vi "Init Scope.vi"(1 "Timeout (ms)":u32=2000, 4 "Scope Control References":T2, 5 "Repetitive Signal":bool, 6 "Reset Settings":bool, 7 "error in (no error)":errorcluster, 8 "Scope Config on Startup":enum16{"PC->Scope", "Scope->PC"}(ring)=enum."Scope->PC", 9 "Scope Model":T1=enum."Tek TDS 694C", 10 "Scope Address":refnum<visa-resource-name>) -> (0 "error out":errorcluster, 2 "Instrument ID":string, 3 "reference out":refnum<visa-resource-name>)   [LabVIEW 2020]
uses:
  Typedefs/Scope Control References Control.ctl
  Typedefs/Scope Models.ctl
  730dcbdf-4df6-4714-a0fe-e75e7198162a.vi
  7d0b5108-51c8-4697-949d-e607a969f50b.vi
  <instrlib>/tktds7xx/tktds7xx.llb/TKTDS 7XX Trigger Mode/Holdoff.vi
  <vilib>/Comparison/Equal/Equal Functor/Equal Functor.lvclass
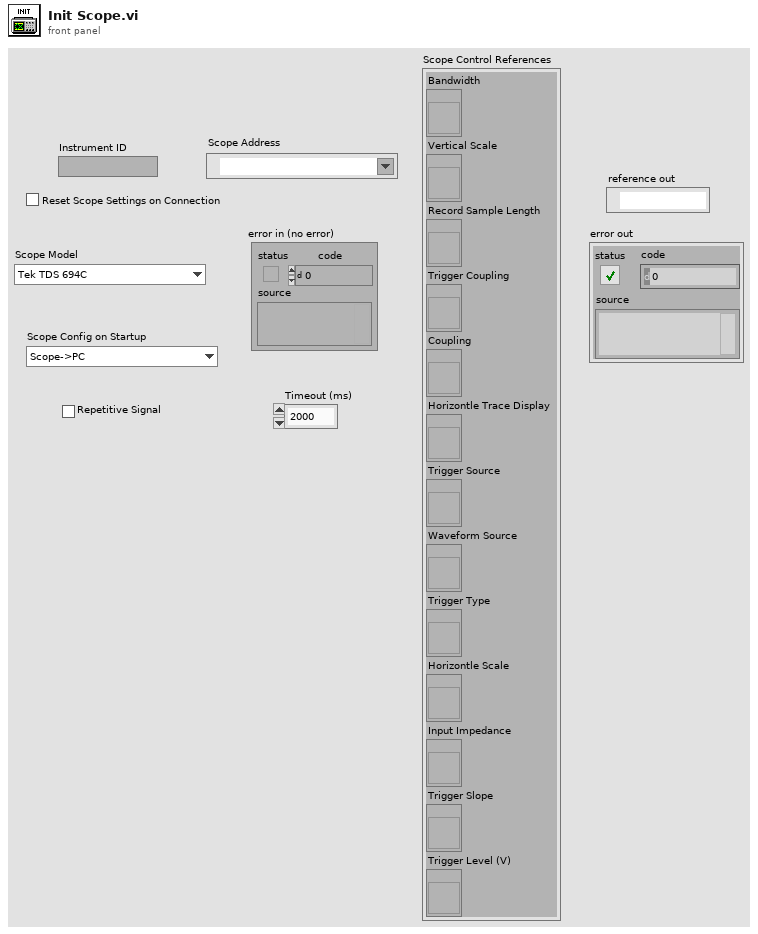
[diagram p1: front panel]
types:
  T1 = typedef "Scope Models.ctl" = enum16{"Tek TDS 684A/B/C", "Tek TDS 694C", "Tek TDS 744/A", "Tek TDS 754A/C/D", "Tek TDS 784A/C/D"}
  T2 = typedef "Scope Control References Control.ctl" = cluster{"Bandwidth":refnum<vi>, "Vertical Scale":refnum<vi>, "Record Sample Length":refnum<vi>, "Trigger Coupling":refnum<vi>, "Coupling":refnum<vi>, "Horizontle Trace Display":refnum<vi>, "Trigger Source":refnum<vi>, "Waveform Source":refnum<vi>, "Trigger Type":refnum<vi>, "Horizontle Scale":refnum<vi>, "Input Impedance":refnum<vi>, "Trigger Slope":refnum<vi>, "Trigger Level (V)":refnum<vi>}
  T3 = cluster{"delay mode (runs after:0)":i32, "delay scaling (50micros/div:16)":i32, "delay events (2)":ext, "delay by (time:0)":i32, "delay time (16.0E-9)":ext}
  T4 = cluster{"Attenuation (Multiplier)":dbl, "Scale (V/Div)":dbl, "Position (V)":dbl, "Offset (V)":dbl, "Coupling":u16, "Impedance":i32, "Bandwidth":i32, "Deskew (s)":dbl}
  T5 = cluster{"Horizontal Mode\n(main only:0)":i32, "Record Length":i32, "Main Scaling (s/Div)":dbl, "Delay Scaling (s/Div)":dbl, "Delay Time (s)":dbl, "Horizontal Position (%)":dbl, "Trigger Position (%)":dbl}
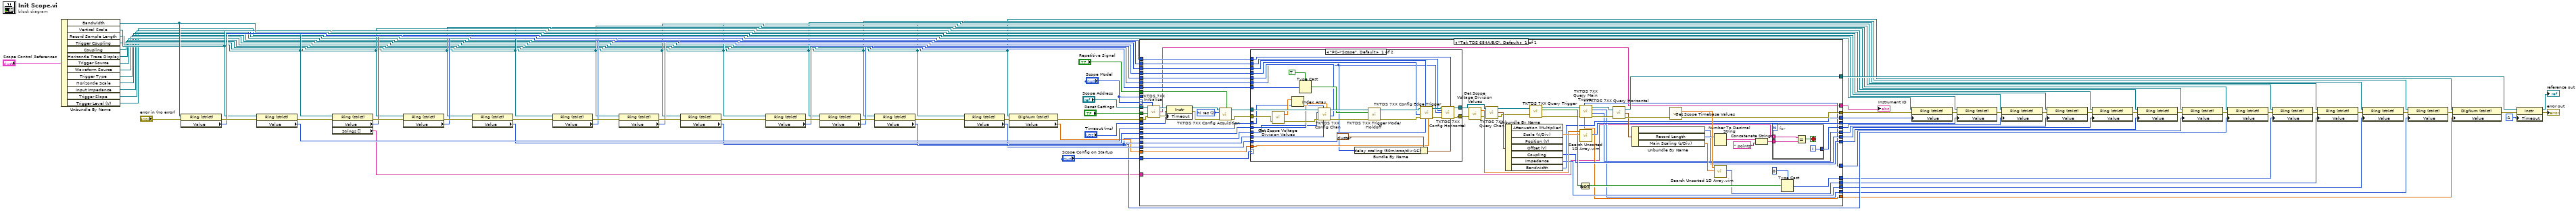
[diagram p0: block diagram]
diagram:
  n1 = Unbundle By Name("Scope Control References") -> ("Bandwidth"=w32:refnum<vi>, "Vertical Scale"=w31:refnum<vi>, "Record Sample Length"=w30:refnum<vi>, "Trigger Coupling"=w29:refnum<vi>, "Coupling"=w28:refnum<vi>, "Horizontle Trace Display"=w27:refnum<vi>, "Trigger Source"=w26:refnum<vi>, "Waveform Source"=w25:refnum<vi>, "Trigger Type"=w24:refnum<vi>, "Horizontle Scale"=w23:refnum<vi>, "Input Impedance"=w22:refnum<vi>, "Trigger Slope"=w21:refnum<vi>, "Trigger Level (V)"=w20:refnum<vi>)
  n2 = property on="Property Node" class="Ring (strict)"(reference=w32, error in="error in (no error)") -> (error out=w75:errorcluster, "Value"=w62:u16)  [unwired: 1 out]
  n3 = property on="Property Node" class="Ring (strict)"(reference=w31, error in=w75) -> (error out=w74:errorcluster, "Value"=w63:u16)  [unwired: 1 out]
  n4 = property on="Property Node" class="Ring (strict)"(reference=w30, error in=w74) -> (error out=w73:errorcluster, "Value"=w54:i32, "Strings []"=w6:string[])  [unwired: 1 out]
  n5 = property on="Property Node" class="Ring (strict)"(reference=w29, error in=w73) -> (error out=w72:errorcluster, "Value"=w56:i32)  [unwired: 1 out]
  n6 = property on="Property Node" class="Ring (strict)"(reference=w28, error in=w72) -> (error out=w71:errorcluster, "Value"=w61:u16)  [unwired: 1 out]
  n7 = property on="Property Node" class="Ring (strict)"(reference=w27, error in=w71) -> (error out=w70:errorcluster, "Value"=w53:i32)  [unwired: 1 out]
  n8 = property on="Property Node" class="Ring (strict)"(reference=w26, error in=w70) -> (error out=w69:errorcluster, "Value"=w55:u16)  [unwired: 1 out]
  n9 = property on="Property Node" class="Ring (strict)"(reference=w25, error in=w69) -> (error out=w68:errorcluster, "Value"=w12:u16)  [unwired: 1 out]
  n10 = property on="Property Node" class="Ring (strict)"(reference=w24, error in=w68) -> (error out=w67:errorcluster, "Value"=w59:u16)  [unwired: 1 out]
  n11 = property on="Property Node" class="Ring (strict)"(reference=w23, error in=w67) -> (error out=w66:errorcluster, "Value"=w52:i32)  [unwired: 1 out]
  n12 = property on="Property Node" class="Ring (strict)"(reference=w22, error in=w66) -> (error out=w65:errorcluster, "Value"=w60:u16)  [unwired: 1 out]
  n13 = property on="Property Node" class="Ring (strict)"(reference=w21, error in=w65) -> (error out=w64:errorcluster, "Value"=w58:i32)  [unwired: 1 out]
  n14 = property on="Property Node" class="DigNum (strict)"(reference=w20, error in=w64) -> (error out=w3:errorcluster, "Value"=w57:dbl)  [unwired: 1 out]
  n15 = case shown="\"Tek TDS 684A/B/C\", Default" "Scope Model" {
    selector: "Scope Model" -> [w81]
    tunnel: "Scope Model" -> [_]
    tunnel: "Repetitive Signal" -> [w144]
    tunnel: "Scope Config on Startup" -> [w143]
    tunnel: "Scope Address" -> [w139]
    tunnel: "Reset Settings" -> [w138]
    tunnel: w63 -> [w137]
    tunnel: w62 -> [w136]
    tunnel: w61 -> [w135]
    tunnel: w60 -> [w134]
    tunnel: w59 -> [w133]
    tunnel: w58 -> [w132]
    tunnel: w57 -> [w131]
    tunnel: w56 -> [w130]
    tunnel: w55 -> [w129]
    tunnel: w54 -> [w128]
    tunnel: w53 -> [w127]
    tunnel: w52 -> [w126]
    tunnel: [w103] -> w49
    tunnel: "Timeout (ms)" -> [w102]
    tunnel: [w101] -> w35
    tunnel: [w100] -> w19
    tunnel: [w99] -> w18
    tunnel: [w98] -> w17
    tunnel: [w97] -> w16
    tunnel: [w96] -> w15
    tunnel: [w95] -> w14
    tunnel: [w94] -> w13
    tunnel: w12 -> [w93]
    tunnel: [w92] -> w11
    tunnel: [w91] -> w10
    tunnel: [w90] -> w9
    tunnel: [w89] -> w8
    tunnel: [w88] -> w7
    tunnel: w6 -> [w87]
    tunnel: w3 -> [w83]
    tunnel: [w80] -> w1
    frame "Tek TDS 684A/B/C", Default {
      w145 = 2 items=["sample", "peak detect", "hi res", "envelope", "average"] ("acqusition mode (0:sample)")
      n16 = call <instrlib>:"TKTDS 7XX Initialize.vi"("instrument descriptor (GPIB::2)"=w139, "reset"=w138, "error in (no error)"=w83, "model"=w81) -> ("VISA session"=w86:refnum<visa-resource-name>, "Instrument ID"=w80:string, "error out"=w142:errorcluster)  [unwired: 1 in]
      n17 = property class="Instr"(reference=w86, error in=w142, "Timeout"=w102) -> (reference out=w85:refnum<visa-resource-name>, error out=w141:errorcluster)
      n18 = call <instrlib>:"TKTDS 7XX Config Acquisition.vi"("error in (no error)"=w141, "acqusition mode (0:sample)"=w145, "VISA session"=w85, "repetitive signal (T:on)"=w144) -> ("error out"=w82:errorcluster, "dup VISA session"=w140:refnum<visa-resource-name>)  [unwired: 4 in]
      n19 = case shown="\"PC->Scope\", Default" w143 {
        tunnel: w82 -> [w173 w181]
        tunnel: w140 -> [w170 w180]
        tunnel: w137 -> [w165 _]
        tunnel: w136 -> [w164 _]
        tunnel: w135 -> [w163 _]
        tunnel: w93 -> [w159 _]
        tunnel: w134 -> [w162 _]
        tunnel: w133 -> [w161 _]
        tunnel: w132 -> [w158 _]
        tunnel: w131 -> [w157 _]
        tunnel: w130 -> [w156 _]
        tunnel: w129 -> [w155 _]
        tunnel: w128 -> [w154 _]
        tunnel: w127 -> [w153 _]
        tunnel: w126 -> [w152 _]
        tunnel: [w151 w181] -> w105
        tunnel: [w150 w180] -> w104
        frame "PC->Scope", Default {
          n20 = call "Get Scope Voltage Division Values.vi"("error in (no error)"=w173) -> ("error out"=w167:errorcluster, "Volts Per Division Values Array"=w166:dbl[])  [unwired: 1 in]
          n21 = Index Array(array=w166, index=w165) -> (element=w174:dbl)
          n22 = Type Cast(type=TRUE, x=w161) -> (*(type *) &x=w175:bool)
          n23 = call <instrlib>:"TKTDS 7XX Config Chan.vi"("bandwidth (20MHz:0)"=w164, "scaling (1.0)"=w174, "impedance (50ohms:0)"=w162, "coupling (DC:1)"=w163, "error in (no error)"=w167, "channel to set (ch1:0)"=w159, "VISA session"=w170) -> ("error out"=w160:errorcluster, "dup VISA session"=w177:refnum<visa-resource-name>)  [unwired: 2 in, 1 out]
          n24 = Bundle By Name(cluster=T3 {"delay mode (runs after:0)"=0, "delay scaling (50micros/div:16)"=18, "delay events (2)"=2.0, "delay by (time:0)"=0, "delay time (16.0E-9)"=1.6e-08}, "delay scaling (50micros/div:16)"=w152) -> (w178:T3)
          n25 = call "TKTDS 7XX Trigger Mode/Holdoff.vi"("error in (no error)"=w160, "trigger mode (T:auto)"=w175, "VISA session"=w177) -> ("error out"=w172:errorcluster, "dup VISA session"=w169:refnum<visa-resource-name>)  [unwired: 6 in, 1 out]
          n26 = call <instrlib>:"TKTDS 7XX Config Edge Trigger.vi"("voltage level"=w157, "trigger slope (pos:0)"=w158, "trigger coupling (DC:1)"=w156, "error in (no error)"=w172, "trigger source (ch1:0)"=w155, "VISA session"=w169) -> ("error out"=w171:errorcluster, "dup VISA session"=w168:refnum<visa-resource-name>)  [unwired: 4 in]
          n27 = call <instrlib>:"TKTDS 7XX Config Horizontal.vi"("VISA session"=w168, "record length (500:0)"=w154, "horizontal mode\n(main only:0)"=w153, "main scaling\n(500ps:1)"=w152, "error in (no error)"=w171, 14:w178) -> ("dup VISA session"=w150:refnum<visa-resource-name>, "error out"=w151:errorcluster)  [unwired: 8 in]
        }
        frame "Scope->PC" {
        }
      }
      n28 = call "Get Scope Voltage Division Values.vi"("error in (no error)"=w105) -> ("error out"=w84:errorcluster, "Volts Per Division Values Array"=w125:dbl[])  [unwired: 1 in]
      n29 = call <instrlib>:"TKTDS 7XX Query Chan.vi"("error in (no error)"=w84, "VISA session"=w104) -> ("error out"=w111:errorcluster, "Channel Settings Cluster"=w115:T4, "dup VISA session"=w108:refnum<visa-resource-name>)  [unwired: 1 in]
      n30 = Unbundle By Name(w115) -> ("Scale (V/Div)"=w118:dbl, "Coupling"=w96:u16, "Impedance"=w90:i32, "Bandwidth"=w100:i32)  [unwired: 3 out]
      n31 = call <instrlib>:"TKTDS 7XX Query Trigger.vi"("VISA session"=w108, "error in (no error)"=w111) -> ("dup VISA session"=w109:refnum<visa-resource-name>, "Auto Trigger?"=w116:bool, "error out"=w112:errorcluster)  [unwired: 1 out]
      n32 = Not(x=w116) -> (.not. x?=w117:bool)
      n33 = call <instrlib>:"TKTDS 7XX Query Main Trigger.vi"("error in (no error)"=w112, "VISA session"=w109) -> ("error out"=w113:errorcluster, "Trigger Coupling"=w97:i32, "Trigger Slope"=w89:i32, "dup VISA session"=w110:refnum<visa-resource-name>, "Trigger Level (V)"=w88:dbl, "Trigger Source"=w94:i32)  [unwired: 2 in]
      n34 = call "Search Unsorted 1D Array.vim"("element"=w118, "unsorted 1D array"=w125) -> ("index of element"=w99:i32)  [unwired: 9 in]
      n35 = call <instrlib>:"TKTDS 7XX Query Horizontal.vi"("VISA session"=w110, "error in (no error)"=w113) -> ("dup VISA session"=w103:refnum<visa-resource-name>, "Horizontal Settings"=w114:T5, "error out"=w124:errorcluster)
      n36 = Unbundle By Name(w114) -> ("Horizontal Mode\n(main only:0)"=w95:i32, "Record Length"=w120:i32, "Main Scaling (s/Div)"=w119:dbl)
      n37 = call "Get Scope Timebase Values.vi"("error in (no error)"=w124) -> ("error out"=w101:errorcluster, "Timebase Values Array"=w123:dbl[])  [unwired: 1 in]
      n38 = Number To Decimal String(number=w120) -> (decimal integer string=w121:string)  [unwired: 1 in]
      n39 = call "Search Unsorted 1D Array.vim"("element"=w119, "unsorted 1D array"=w123) -> ("index of element"=w91:i32)  [unwired: 9 in]
      n40 = Concatenate Strings(w121, " points" ("string")) -> (w122:string)
      n41 = for {
        tunnel: w87 -> [w149] mode=indexing
        tunnel: w122 -> [w148]
        tunnel: [w146] -> w98
        i -> [w146]
        stop <- w147 stop-if-true
        n42 = Equal?(x=w149, y=w148) -> (x = y?=w147:bool)
      }
      n43 = Type Cast(type=0, x=w117) -> (*(type *) &x=w92:i32)
    }
  }
  "Instrument ID" <- w1
  n44 = property on="Property Node" class="Ring (strict)"(reference=w32, error in=w35, "Value"=w19) -> (error out=w47:errorcluster)  [unwired: 1 out]
  n45 = property on="Property Node" class="Ring (strict)"(reference=w31, error in=w47, "Value"=w18) -> (error out=w46:errorcluster)  [unwired: 1 out]
  n46 = property on="Property Node" class="Ring (strict)"(reference=w30, error in=w46, "Value"=w17) -> (error out=w45:errorcluster)  [unwired: 1 out]
  n47 = property on="Property Node" class="Ring (strict)"(reference=w29, error in=w45, "Value"=w16) -> (error out=w44:errorcluster)  [unwired: 1 out]
  n48 = property on="Property Node" class="Ring (strict)"(reference=w28, error in=w44, "Value"=w15) -> (error out=w43:errorcluster)  [unwired: 1 out]
  n49 = property on="Property Node" class="Ring (strict)"(reference=w27, error in=w43, "Value"=w14) -> (error out=w42:errorcluster)  [unwired: 1 out]
  n50 = property on="Property Node" class="Ring (strict)"(reference=w26, error in=w42, "Value"=w13) -> (error out=w41:errorcluster)  [unwired: 1 out]
  n51 = property on="Property Node" class="Ring (strict)"(reference=w25, error in=w41, "Value"=w12) -> (error out=w40:errorcluster)  [unwired: 1 out]
  n52 = property on="Property Node" class="Ring (strict)"(reference=w24, error in=w40, "Value"=w11) -> (error out=w39:errorcluster)  [unwired: 1 out]
  n53 = property on="Property Node" class="Ring (strict)"(reference=w23, error in=w39, "Value"=w10) -> (error out=w38:errorcluster)  [unwired: 1 out]
  n54 = property on="Property Node" class="Ring (strict)"(reference=w22, error in=w38, "Value"=w9) -> (error out=w37:errorcluster)  [unwired: 1 out]
  n55 = property on="Property Node" class="Ring (strict)"(reference=w21, error in=w37, "Value"=w8) -> (error out=w36:errorcluster)  [unwired: 1 out]
  n56 = property on="Property Node" class="DigNum (strict)"(reference=w20, error in=w36, "Value"=w7) -> (error out=w34:errorcluster)  [unwired: 1 out]
  n57 = property class="Instr"(reference=w49, error in=w34, "Timeout"=-1) -> (reference out=→"reference out":refnum<visa-resource-name>, error out=→"error out":errorcluster)
